vi "savePath.vi"(8 "error in (no error)":errorcluster, 9 "overwrite?":bool, 10 "Path  in":path) -> (0 "error out":errorcluster, 1 "cancelled":bool, 2 "Path out":path)   [LabVIEW 2011, in "Views.lvlib" / "SettingsViewer.lvclass"]
uses:
  settingsViewer.lvclass
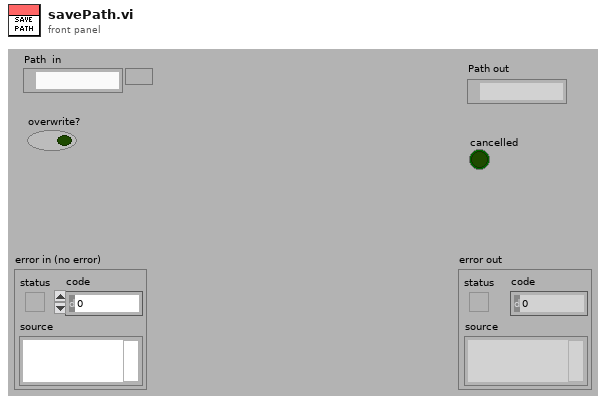
[diagram p1: front panel]
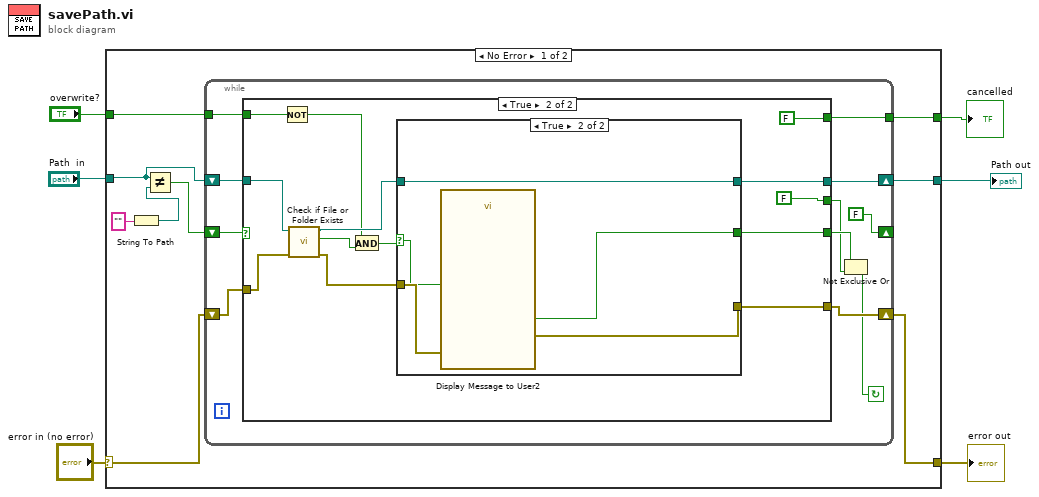
[diagram p0: block diagram]
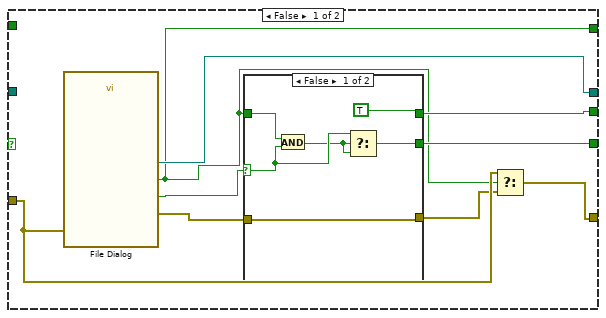
[diagram p2: hidden frame]
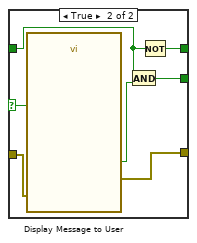
[diagram p3: hidden frame]
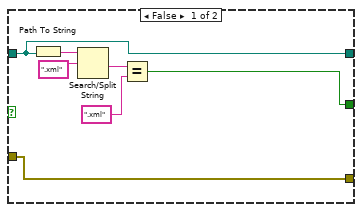
[diagram p4: hidden frame]
diagram:
  n1 = case shown="No Error" "error in (no error)" {
    selector: "error in (no error)" -> [w9 w75]
    tunnel: [w10 w75] -> w5
    tunnel: "Path  in" -> [w12 w74]
    tunnel: [w11 w74] -> w3
    tunnel: "overwrite?" -> [w8 _]
    tunnel: [w7 _] -> w1
    frame No Error {
      n2 = String To Path(string="") -> (path=w13:path)
      n3 = Not Equal?(x=w12, y=w13) -> (x != y?=w14:bool)
      n4 = while {
        shift-right: [w22] -> w11
        shift-left: w12 -> [w21]
        shift-right: [FALSE] -> _
        shift-left: w14 -> [w26]
        shift-right: [w24] -> w10
        shift-left: w9 -> [w25]
        tunnel: w8 -> [w17]
        tunnel: [w16] -> w7
        stop <- w19 continue-if-true
        n5 = case shown="True" w26 {
          tunnel: w25 -> [w31 w56]
          tunnel: [w33 w61] -> w24
          tunnel: [w32 w55] -> w23
          tunnel: [w34 w60] -> w22
          tunnel: w21 -> [_ w59]
          tunnel: [w29 FALSE] -> w18
          tunnel: w17 -> [_ w51]
          tunnel: [w27 FALSE] -> w16
          frame False {
            n6 = call "File Dialog"("error in"=w31) -> ("selected path"=w34:path, "exists"=w28:bool, "cancelled"=w27:bool, "error out"=w35:errorcluster)  [unwired: 11 in]
            n7 = case shown="False" w28 {
              selector: w28 -> [w40 w46]
              tunnel: w35 -> [w41 w48]
              tunnel: [w41 w47] -> w30
              tunnel: [w38 w44] -> w32
              tunnel: w27 -> [w37 w43]
              tunnel: [TRUE w42] -> w29
              frame False {
                n8 = And(x=w37, y=w40) -> (x .and. y?=w39:bool)
                n9 = Select(t=w40, s=w39, f=w39) -> (s? t:f=w38:bool)
              }
              frame True {
                n10 = call "Display Message to User"("error in (no error)"=w48, "Enable"=w46) -> ("error out"=w47:errorcluster, "Overwrite"=w45:bool)  [unwired: 8 in]
                n11 = And(x=w43, y=w45) -> (x .and. y?=w44:bool)
                n12 = Not(x=w43) -> (.not. x?=w42:bool)
              }
            }
            n13 = Select(t=w31, s=w27, f=w30) -> (s? t:f=w33:errorcluster)
          }
          frame True {
            n14 = Not(x=w51) -> (.not. x?=w50:bool)
            n15 = call <vilib>:"Check if File or Folder Exists.vi"("error in (no error)"=w56, "path"=w59) -> ("error out"=w57:errorcluster, "file or folder exists?"=w52:bool, "dup path"=w58:path)  [unwired: 7 in]
            n16 = And(x=w50, y=w52) -> (x .and. y?=w53:bool)
            n17 = case shown="True" w53 {
              selector: w53 -> [_ w70]
              tunnel: w57 -> [w68 w73]
              tunnel: w58 -> [w64 w71]
              tunnel: [w64 w71] -> w60
              tunnel: [w68 w72] -> w61
              tunnel: [w63 w69] -> w55
              frame False {
                n18 = Path To String(path=w64) -> (string=w67:string)
                n19 = Search/Split String(string=w67, search string/char (-)=".xml") -> (match + rest of string=w65:string)  [unwired: 1 in, 2 out]
                n20 = Equal?(x=w65, y=".xml") -> (x = y?=w63:bool)
              }
              frame True {
                n21 = call "Display Message to User2"("error in (no error)"=w73, "Enable"=w70) -> ("error out"=w72:errorcluster, "Overwrite"=w69:bool)  [unwired: 8 in]
              }
            }
          }
        }
        n22 = Not Exclusive Or(1:w18, 2:w23) -> (0:w19:bool)
      }
    }
    frame Error {
    }
  }
  "error out" <- w5
  "Path out" <- w3
  "cancelled" <- w1
